vi "Change Setpoint.vi"(8 "error in (no error)":errorcluster, 10 "Setpoint":dbl, 11 "MFC in":refnum<class "MFC.lvclass">) -> (0 "error out":errorcluster, 3 "MFC out":refnum<class "MFC.lvclass">)   [LabVIEW 2018, in "MFC Actor.lvlib" / "MFC.lvclass"]
uses:
  MFC.lvclass
  C:/Program Files/National Instruments/LabVIEW 2018/vi.lib/ActorFramework/Actor/Actor.lvclass
  MFC.lvclass/MFC.ctl
  <vilib>/ActorFramework/Actor/Actor.lvclass/Actor.ctl
  ADM/Main Messages/Switch Solenoid Feedthrough Msg/Switch Solenoid Feedthrough Msg.lvclass/Switch Solenoid Feedthrough Msg.ctl
  <vilib>/ActorFramework/Message Enqueuer/Message Enqueuer.lvclass/Message Enqueuer.ctl
  <vilib>/ActorFramework/Message Enqueuer/Enqueue.vi
  ADM/Main Messages/Switch Solenoid Feedthrough Msg/Switch Solenoid Feedthrough Msg.lvclass
  C:/Program Files/National Instruments/LabVIEW 2018/vi.lib/ActorFramework/Message/Message.lvclass
  <vilib>/ActorFramework/Message Priority Queue/Priority Enqueue.vi
  <instrlib>/Sierra Instruments Smart-Trak 100 Series/Sierra Instruments Smart-Trak 100 Series.lvlib
  <vilib>/ActorFramework/Actor/Actor.lvclass
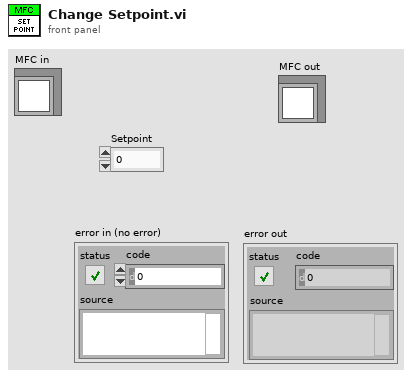
[diagram p1: front panel]
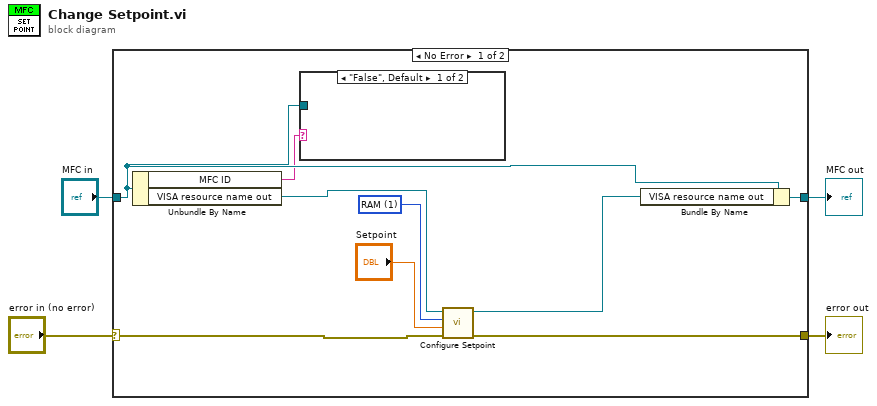
[diagram p0: block diagram]
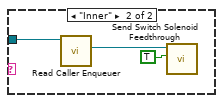
[diagram p2: hidden frame]
diagram:
  n1 = case shown="No Error" "error in (no error)" {
    selector: "error in (no error)" -> [w9 w17]
    tunnel: [w13 w18] -> w1
    tunnel: [w12 w17] -> w4
    tunnel: "MFC in" -> [w11 w18]
    frame No Error {
      w6 = u16 1 items=["Flash", "RAM"] ("Memory Type (0: Flash)")
      n2 = Unbundle By Name(w11) -> ("MFC ID"=w8:string, "VISA resource name out"=w7:refnum<visa-resource-name>)
      n3 = case shown="\"False\", Default" w8 {
        tunnel: w11 -> [_ w16]
        frame "False", Default {
        }
        frame "Inner" {
          n4 = call <vilib>:"Read Caller Enqueuer.vi"("Actor"=w16) -> ("Caller Enqueuer"=w15:refnum<class "Message Enqueuer.lvclass">)  [unwired: 10 in]
          n5 = call "Send Switch Solenoid Feedthrough.vi"("Only Turn On (F)"=TRUE, "Message Enqueuer"=w15) -> ()  [unwired: 8 in, 2 out]
        }
      }
      n6 = call <instrlib>:"Configure Setpoint.vi"("error in (no error)"=w9, "Setpoint Value (0)"="Setpoint", "Memory Type (0: Flash)"=w6, "VISA resource name"=w7) -> ("error out"=w12:errorcluster, "VISA resource name out"=w10:refnum<visa-resource-name>)  [unwired: 6 in]
      n7 = Bundle By Name(cluster=w11, "VISA resource name out"=w10) -> (w13:refnum<class "MFC.lvclass">)
    }
    frame Error {
    }
  }
  "error out" <- w4
  "MFC out" <- w1
